vi "Test Slave API.vi"() -> ()   [LabVIEW 2021, in "Slave.lvlib"]
doc: "Slave API Tester.\n\n<b>Note:</b> This VI was modified by the <b>Validate DQMH Module</b> tool to remove code to stop the main loop on error, and instead display the most recent error on the tester front panel."
uses:
  <vilib>/Utility/error.llb/DialogType.ctl
  Slave.lvlib
panel:
  out "last error":errorcluster
  out "Title":string
  in  "Show Diagram on Init":bool
  in  "Run as Singleton?":bool
  in  "Show Block Diagram":bool
  in  "Refresh Modules":bool
  out "Active Modules":string[](array[string])
  in  "Stop Module":bool
  in  "Select Module":i32(ring)=-1 caption="Select Module\nTo send Request to" items=["All"=-1]
  in  "Run New Module":bool
  in  "Hide Module Panel":bool
  in  "Show Module Panel":bool
  out "Status":string
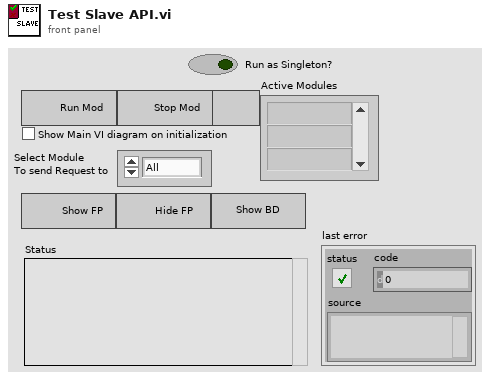
[diagram p1: front panel]
types:
  T1 = typedef "Slave.lvlib/Broadcast Events--cluster.ctl" = cluster{"Module Did Init":refnum<user-event>, "Status Updated":refnum<user-event>, "Error Reported":refnum<user-event>, "Module Did Stop":refnum<user-event>, "Update Module Execution Status":refnum<user-event>}
  T2 = typedef "DialogType.ctl" = u16
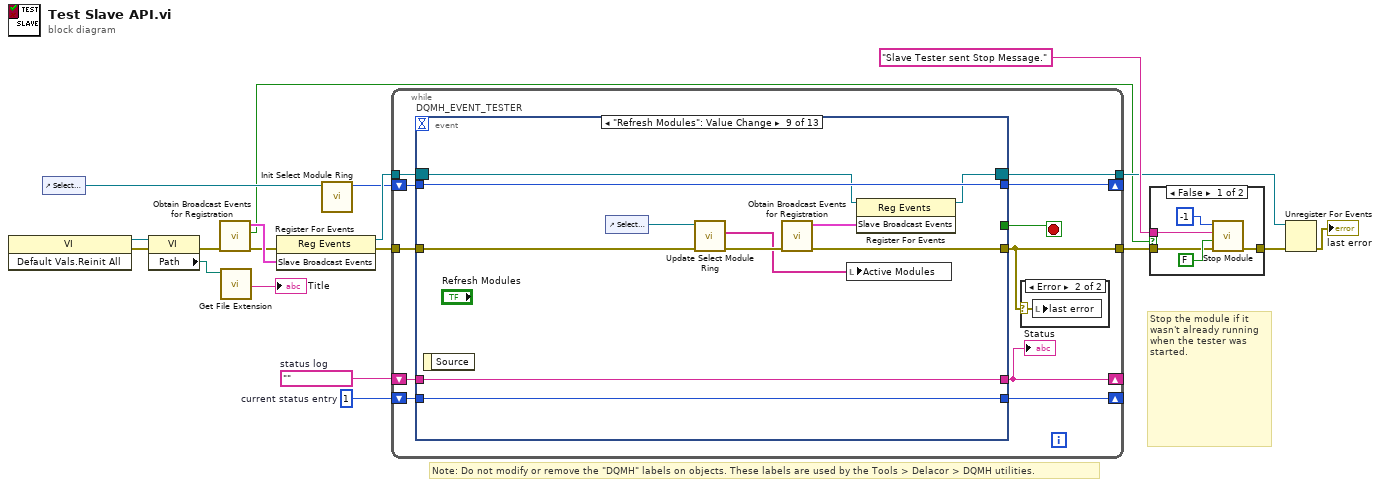
[diagram p0: block diagram]
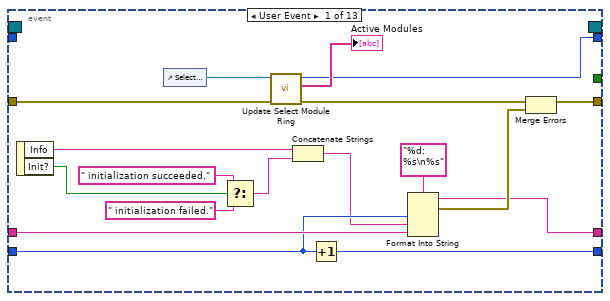
[diagram p4: hidden frame]
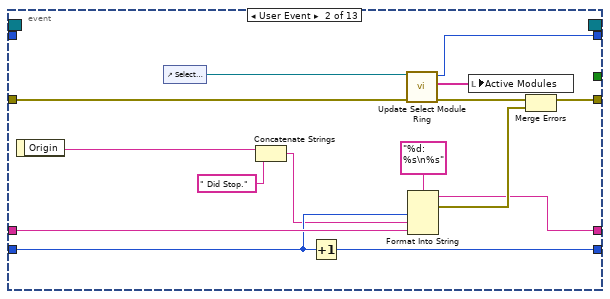
[diagram p5: hidden frame]
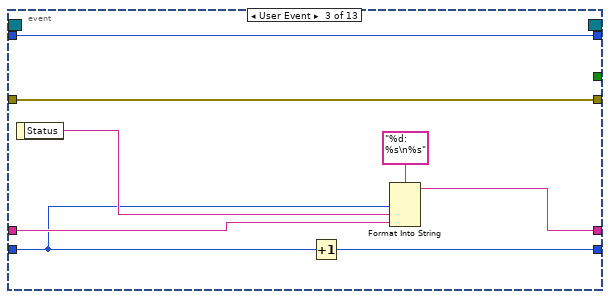
[diagram p6: hidden frame]
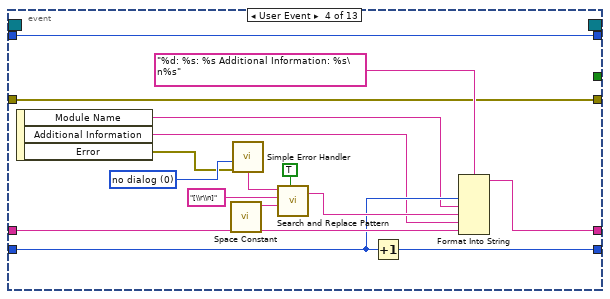
[diagram p7: hidden frame]
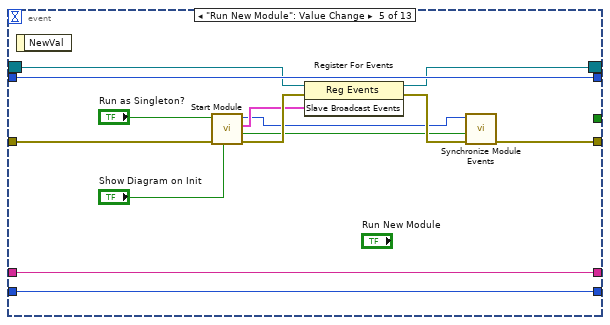
[diagram p8: hidden frame]
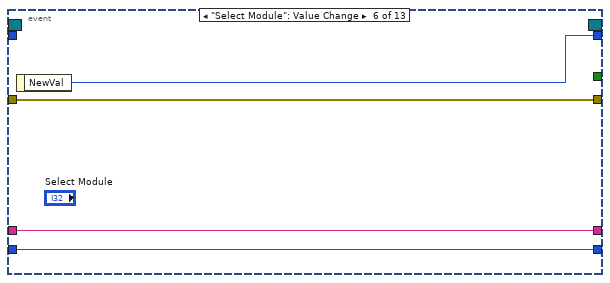
[diagram p9: hidden frame]
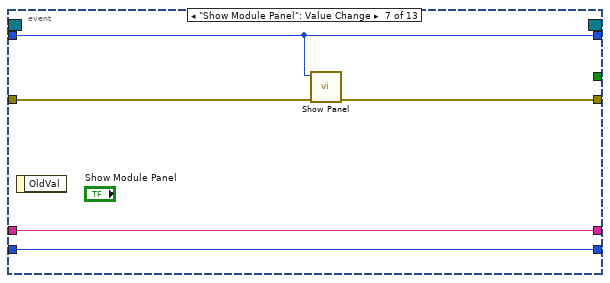
[diagram p10: hidden frame]
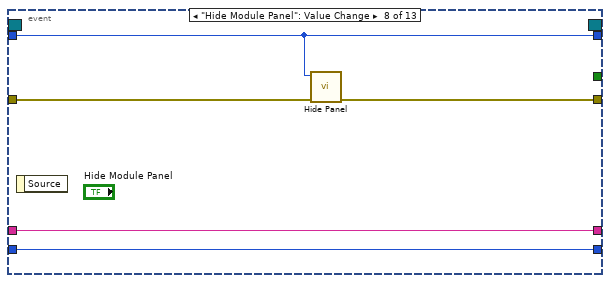
[diagram p11: hidden frame]
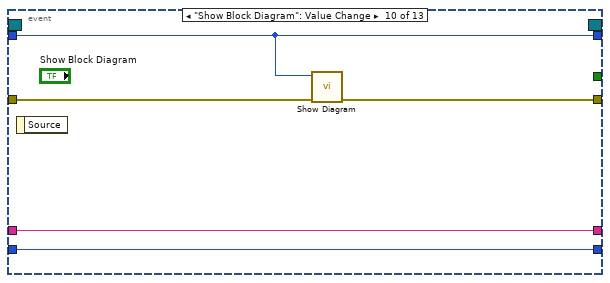
[diagram p12: hidden frame]
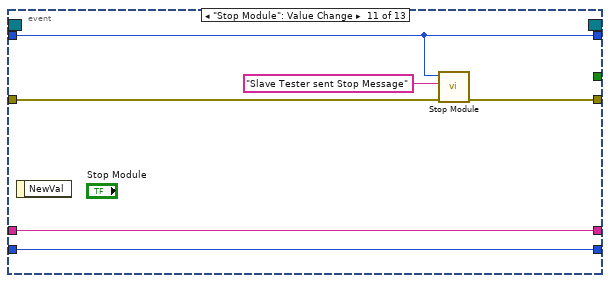
[diagram p13: hidden frame]
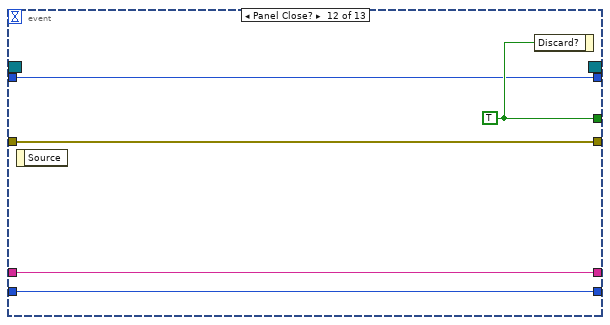
[diagram p14: hidden frame]
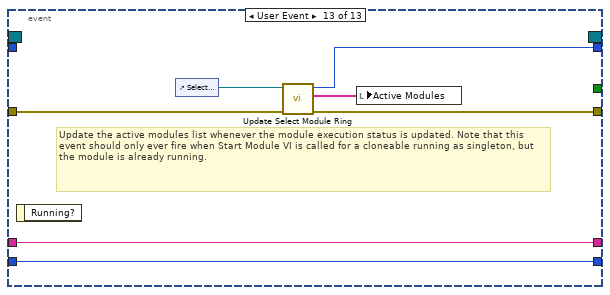
[diagram p15: hidden frame]
diagram:
  w16 = 1  # current status entry
  w17 = ""  # status log
  # "Stop the module if it wasn't already running when the tester was started."
  # "Note: Do not modify or remove the \"DQMH\" labels on objects. These labels are used by the Tools > Delacor > DQMH utilities."
  n1 = invoke class="VI" method="Default Vals.Reinit All"() -> (reference out=w3:refnum<vi>, error out=w9:errorcluster)  [unwired: 3 in, 1 out]
  n2 = control-ref of="Select Module"() -> (w14:refnum<vi>)
  n3 = property class="VI"(reference=w3, error in=w9) -> (error out=w4:errorcluster, "Path"=w2:path)  [unwired: 1 out]
  n4 = call "Obtain Broadcast Events for Registration.vi"("error in"=w4) -> ("error out"=w8:errorcluster, "Already running?"=w7:bool, "Slave Broadcast Events"=w13:T1)  [unwired: 8 in]
  n5 = call <vilib>:"Get File Extension.vi"("file"=w2) -> ("filename without extension"=→"Title":string)  [unwired: 6 in, 4 out]
  n6 = register-events(error in=w8, w13) -> (reference out=w19:refnum<event-registration>, error out=w12:errorcluster)  [unwired: 1 in]
  n7 = call "Init Select Module Ring.vi"("Select Module Ring Ref"=w14) -> ("Value for All Modules"=w15:i32)  [unwired: 8 in, 2 out]
  n8 = while {
    tunnel: w19 -> [w30]
    tunnel: [w21] -> w6
    tunnel: w12 -> [w29]
    shift-right: [w25] -> _
    shift-left: w17 -> [w27]
    shift-right: [w26] -> _
    shift-left: w16 -> [w28]
    shift-right: [w23] -> _
    shift-left: w15 -> [w24]
    tunnel: [w22] -> w10
    stop <- w20 stop-if-true
    n9 = event "DQMH_EVENT_TESTER" shown="[8] \"Refresh Modules\": Value Change" {
      selector: w30 -> [_ _ _ _ w96 _ _ _ w122 _ _ _ _]
      dyn-events: [_ _ _ _ w95 _ _ _ w121 _ _ _ _] -> w22
      timeout: _ -> [_ _ _ _ _ _ _ _ _ _ _ _ _]
      tunnel: [_ _ _ _ _ _ _ _ _ _ _ w143 _] -> w20
      tunnel: [w39 w56 w72 w76 w94 w106 w110 w115 w118 w129 w134 w142 w146] -> w21
      tunnel: w29 -> [w41 w58 w72 w76 w97 w106 w111 w116 w123 w132 w135 w142 w147]
      tunnel: w28 -> [w46 w61 w65 w79 w99 w104 w108 w113 w126 w130 w137 w140 w149]
      tunnel: w27 -> [w47 w62 w68 w80 w100 w105 w109 w114 w127 w131 w138 w141 w150]
      tunnel: [w44 w59 w69 w78 w100 w105 w109 w114 w127 w131 w138 w141 w150] -> w25
      tunnel: [w45 w60 w71 w77 w99 w104 w108 w113 w126 w130 w137 w140 w149] -> w26
      tunnel: w24 -> [_ _ w66 w88 w98 _ w107 w112 w125 w128 w136 w139 _]
      tunnel: [w36 w53 w66 w88 w98 w103 w107 w112 w125 w128 w136 w139 w145] -> w23
      event User Event {
        n10 = event-data() -> ("Info"=w43:string, "Init?"=w33:bool)  [unwired: 1 in]
        n11 = control-ref of="Select Module"() -> (w38:refnum<vi>)
        n12 = Select(t=" initialization succeeded.", s=w33, f=" initialization failed.") -> (s? t:f=w32:string)
        n13 = call "Update Select Module Ring.vi"("error in (no error)"=w41, "Select Module Ring Ref"=w38) -> ("error out"=w40:errorcluster, "Active Modules (Array)"=→"Active Modules":string[], "New Module Ring Value"=w36:i32)  [unwired: 7 in]
        n14 = Concatenate Strings(w43, w32) -> (w42:string)
        n15 = Increment(x=w46) -> (x+1=w45:i32)
        n16 = Format Into String(format string="%d: %s\n%s", w46, w42, w47) -> (resulting string=w44:string, error out=w49:errorcluster)  [unwired: 2 in]
        n17 = Merge Errors(w40, w49) -> (w39:errorcluster)
      }
      event User Event {
        n18 = event-data() -> ("Origin"=w51:string)  [unwired: 1 in]
        n19 = control-ref of="Select Module"() -> (w55:refnum<vi>)
        n20 = Concatenate Strings(w51, " Did Stop.") -> (w50:string)
        n21 = Increment(x=w61) -> (x+1=w60:i32)
        n22 = call "Update Select Module Ring.vi"("error in (no error)"=w58, "Select Module Ring Ref"=w55) -> ("error out"=w57:errorcluster, "Active Modules (Array)"=w54:string[], "New Module Ring Value"=w53:i32)  [unwired: 7 in]
        n23 = Format Into String(format string="%d: %s\n%s", w61, w50, w62) -> (resulting string=w59:string, error out=w64:errorcluster)  [unwired: 2 in]
        n24 = local write "Active Modules"(w54) -> ()
        n25 = Merge Errors(w57, w64) -> (w56:errorcluster)
      }
      event User Event {
        n26 = event-data() -> ("Status"=w67:string)  [unwired: 1 in]
        n27 = Increment(x=w65) -> (x+1=w71:i32)
        n28 = Format Into String(format string="%d: %s\n%s", w65, w67, w68) -> (resulting string=w69:string)  [unwired: 2 in, 1 out]
      }
      event User Event {
        w81 = T2 0 items=["no dialog", "OK message", "continue or stop message", "OK message + warnings", "continue/stop + warnings"] ("type of dialog (OK msg:1)")
        n29 = event-data() -> ("Module Name"=w75:string, "Additional Information"=w74:string, "Error"=w73:errorcluster)  [unwired: 1 in]
        n30 = call <vilib>:"Space Constant.vi"() -> ("String"=w85:string)
        n31 = call <vilib>:"Simple Error Handler.vi"("type of dialog (OK msg:1)"=w81, "error in (no error)"=w73) -> ("message"=w82:string)  [unwired: 3 in, 4 out]
        n32 = call <vilib>:"Search and Replace Pattern.vi"("string"=w82, "regular expression (\"\")"="[\\r\\n]" ("regular expression (\"\")"), "replace string (\"\")"=w85, "replace all? (F)"=TRUE ("replace all CR/LF with spaces")) -> ("result string"=w83:string)  [unwired: 1 in, 1 out]
        n33 = Increment(x=w79) -> (x+1=w77:i32)
        n34 = Format Into String(format string="%d: %s: %s Additional Information: %s\n%s", w79, w75, w83, w74, w80) -> (resulting string=w78:string)  [unwired: 2 in, 1 out]
      }
      event "Run New Module": Value Change {
        n35 = event-data() -> ()  [unwired: 1 in, 1 out]
        n36 = call "Start Module.vi"("Show Main VI Diagram on Init (F)"="Show Diagram on Init", "error in"=w97, "Run as Singleton? (F)"="Run as Singleton?") -> ("error out"=w101:errorcluster, "Wait for Event Sync?"=w93:bool, "Slave Broadcast Events"=w92:T1, "Module ID"=w89:i32)  [unwired: 5 in]
        n37 = register-events(reference=w96, error in=w101, w92) -> (reference out=w95:refnum<event-registration>, error out=w102:errorcluster)
        n38 = call "Synchronize Module Events.vi"("error in"=w102, "Wait for Event Sync?"=w93, "Module ID in"=w89) -> ("error out"=w94:errorcluster)  [unwired: 7 in, 1 out]
      }
      event "Select Module": Value Change {
        n39 = event-data() -> ("NewVal"=w103:i32)  [unwired: 1 in]
      }
      event "Show Module Panel": Value Change {
        n40 = event-data() -> ()  [unwired: 1 in, 1 out]
        n41 = call "Show Panel.vi"("error in (no error)"=w111, "Module ID"=w107) -> ("error out"=w110:errorcluster)  [unwired: 9 in]
      }
      event "Hide Module Panel": Value Change {
        n42 = event-data() -> ()  [unwired: 1 in, 1 out]
        n43 = call "Hide Panel.vi"("error in (no error)"=w116, "Module ID"=w112) -> ("error out"=w115:errorcluster)  [unwired: 9 in]
      }
      event "Refresh Modules": Value Change {
        n44 = event-data() -> ()  [unwired: 1 in, 1 out]
        n45 = control-ref of="Select Module"() -> (w124:refnum<vi>)
        n46 = call "Update Select Module Ring.vi"("error in (no error)"=w123, "Select Module Ring Ref"=w124) -> ("error out"=w119:errorcluster, "Active Modules (Array)"=w117:string[])  [unwired: 7 in, 1 out]
        n47 = call "Obtain Broadcast Events for Registration.vi"("error in"=w119) -> ("error out"=w118:errorcluster, "Slave Broadcast Events"=w120:T1)  [unwired: 8 in, 1 out]
        n48 = local write "Active Modules"(w117) -> ()
        n49 = register-events(reference=w122, w120) -> (reference out=w121:refnum<event-registration>)  [unwired: 1 in, 1 out]
      }
      event "Show Block Diagram": Value Change {
        n50 = event-data() -> ()  [unwired: 1 in, 1 out]
        n51 = call "Show Diagram.vi"("error in (no error)"=w132, "Module ID"=w128) -> ("error out"=w129:errorcluster)  [unwired: 9 in]
      }
      event "Stop Module": Value Change {
        n52 = event-data() -> ()  [unwired: 1 in, 1 out]
        n53 = call "Stop Module.vi"("error in"=w135, "Origin"="Slave Tester sent Stop Message", "Module ID"=w136) -> ("error out"=w134:errorcluster)  [unwired: 8 in]
      }
      event Panel Close? {
        w143 = TRUE ("Discard?")
        n54 = event-data() -> ()  [unwired: 1 in, 1 out]
        n55 = event-data("Discard?"=w143) -> ()  [unwired: 1 in, 1 out]
      }
      event User Event {
        # "Update the active modules list whenever the module execution status is updated. Note that this event should only ever fire when Start Module VI is called for a cloneable running as singleton, but the module is already running."
        n56 = event-data() -> ()  [unwired: 1 in, 1 out]
        n57 = control-ref of="Select Module"() -> (w148:refnum<vi>)
        n58 = call "Update Select Module Ring.vi"("error in (no error)"=w147, "Select Module Ring Ref"=w148) -> ("error out"=w146:errorcluster, "Active Modules (Array)"=w144:string[], "New Module Ring Value"=w145:i32)  [unwired: 7 in]
        n59 = local write "Active Modules"(w144) -> ()
      }
    }
    "Status" <- w25
    n60 = case "DQMH_TESTER_ERROR_LOCAL" shown="Error" w21 {
      selector: w21 -> [_ w31]
      frame No Error {
      }
      frame Error {
        n61 = local write "last error"(w31) -> ()
      }
    }
  }
  n62 = case shown="False" w7 {
    tunnel: [w155 w156] -> w18
    tunnel: "Slave Tester sent Stop Message." ("Origin") -> [w154 _]
    tunnel: w6 -> [w151 w156]
    frame False {
      n63 = call "Stop Module.vi"("error in"=w151, "Wait for Module to stop? (F)"=FALSE ("Wait for Module to stop?"), "Origin"=w154, "Module ID"=-1 ("Stop all")) -> ("error out"=w155:errorcluster)  [unwired: 7 in]
    }
    frame True {
    }
  }
  n64 = Unregister For Events(event registration refnum=w10, error in=w18) -> (error out=→"last error":errorcluster)
